vi "sumLinesIntoVolume.vi"(8 "error in (no error)":errorcluster, 10 "volumes to assemble":T3(array[cluster]), 11 "assembler status":T2) -> (0 "error out":errorcluster, 2 "volumes to send":T1(array[cluster]), 3 "assembler status out":T2)   [LabVIEW 2010]
uses:
  get write location linear fit.vi
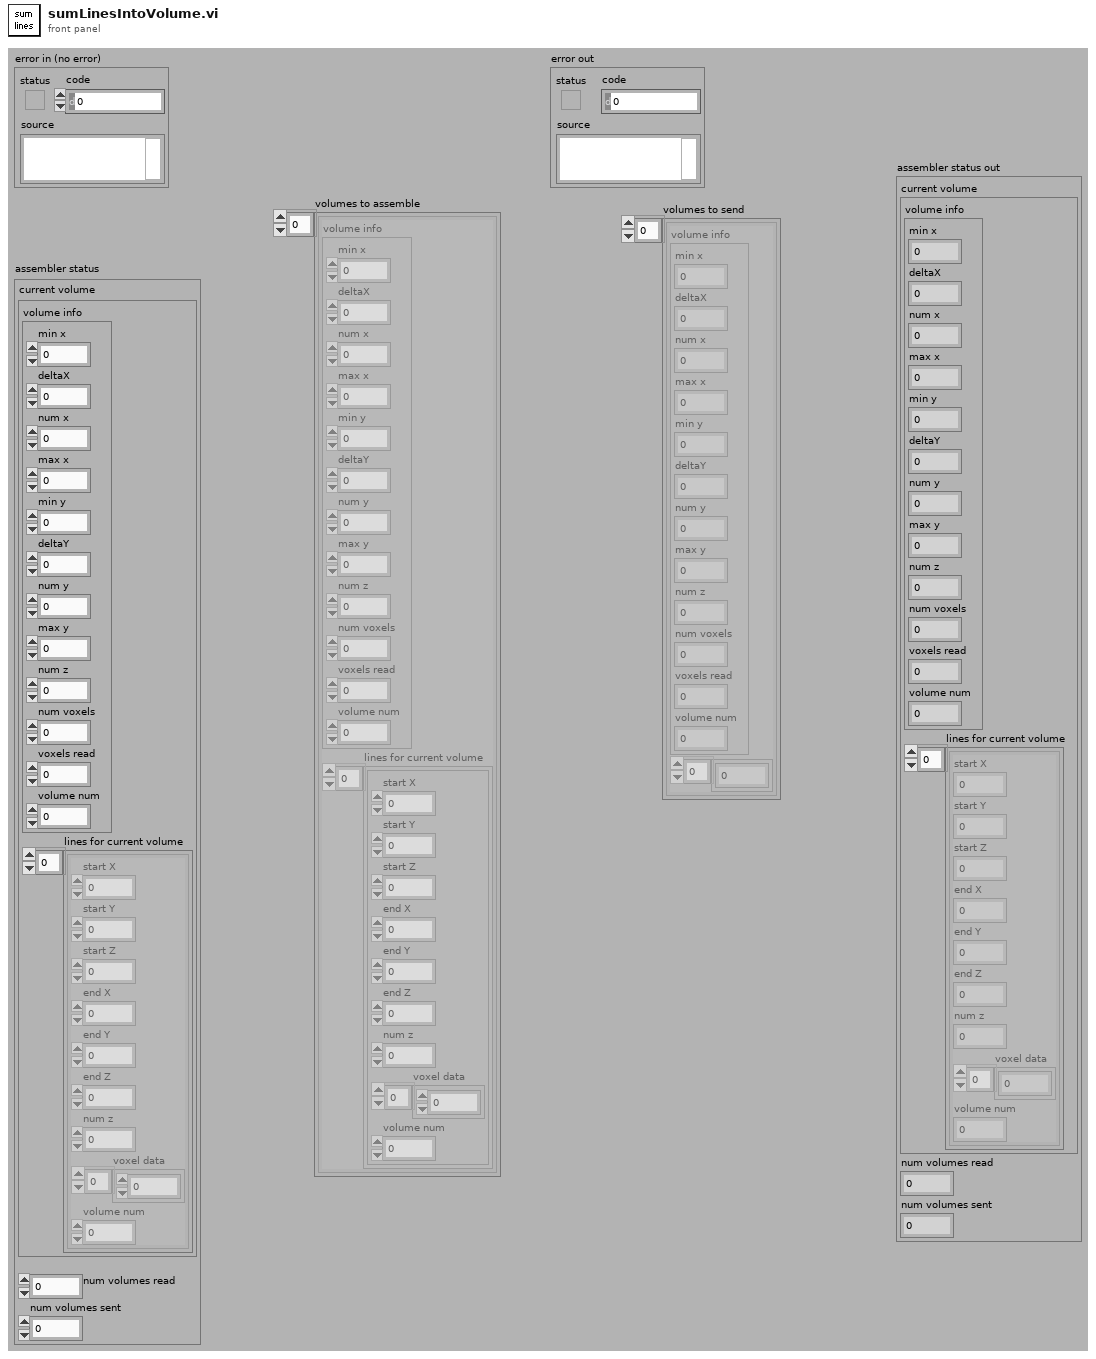
[diagram p1: front panel]
types:
  T1 = cluster{"volume info":cluster{"min x":i16, "deltaX":dbl, "num x":u32, "max x":i16, "min y":i16, "deltaY":dbl, "num y":u32, "max y":i16, "num z":u32, "num voxels":u32, "voxels read":u32, "volume num":u32}, u32[]}[]
  T2 = cluster{"current volume":cluster{"volume info":cluster{"min x":i16, "deltaX":dbl, "num x":u32, "max x":i16, "min y":i16, "deltaY":dbl, "num y":u32, "max y":i16, "num z":u32, "num voxels":u32, "voxels read":u32, "volume num":u32}, "lines for current volume":cluster{"start X":i16, "start Y":i16, "start Z":i16, "end X":i16, "end Y":i16, "end Z":i16, "num z":u8, "voxel data":u32[], "volume num":u32}[]}, "num volumes read":u32, "num volumes sent":u32}
  T3 = cluster{"volume info":cluster{"min x":i16, "deltaX":dbl, "num x":u32, "max x":i16, "min y":i16, "deltaY":dbl, "num y":u32, "max y":i16, "num z":u32, "num voxels":u32, "voxels read":u32, "volume num":u32}, "lines for current volume":cluster{"start X":i16, "start Y":i16, "start Z":i16, "end X":i16, "end Y":i16, "end Z":i16, "num z":u8, "voxel data":u32[], "volume num":u32}[]}[]
  T4 = cluster{"min x":i16, "deltaX":dbl, "num x":u32, "max x":i16, "min y":i16, "deltaY":dbl, "num y":u32, "max y":i16, "num z":u32, "num voxels":u32, "voxels read":u32, "volume num":u32}
  T5 = cluster{"start X":i16, "start Y":i16, "start Z":i16, "end X":i16, "end Y":i16, "end Z":i16, "num z":u8, "voxel data":u32[], "volume num":u32}[]
  T6 = cluster{"volume info":cluster{"min x":i16, "deltaX":dbl, "num x":u32, "max x":i16, "min y":i16, "deltaY":dbl, "num y":u32, "max y":i16, "num z":u32, "num voxels":u32, "voxels read":u32, "volume num":u32}, u32[]}
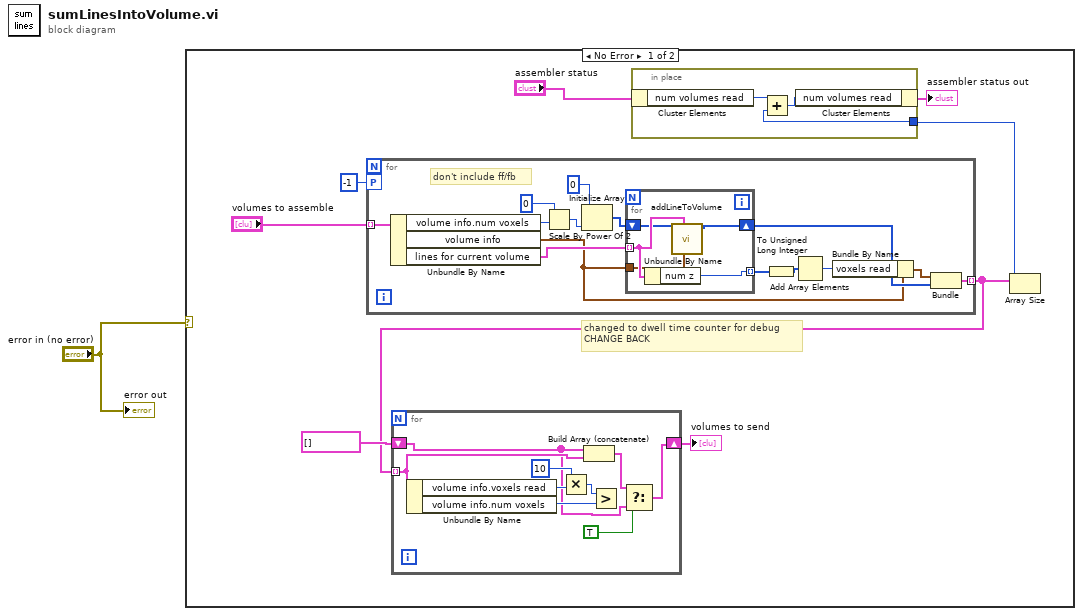
[diagram p0: block diagram]
diagram:
  n1 = case shown="No Error" "error in (no error)" {
    frame No Error {
      # "changed to dwell time counter for debug\nCHANGE BACK"
      n2 = for {
        tunnel: "volumes to assemble" -> [w35] mode=indexing
        tunnel: [w23] -> w6 mode=indexing
        workers-P: -1 -> [_]
        # "don't include ff/fb"
        n3 = Unbundle By Name(w35) -> ("volume info.num voxels"=w34:u32, "volume info"=w24:T4, "lines for current volume"=w29:T5)
        n4 = Scale By Power Of 2(n=0, x=w34) -> (x*2^n=w32:u32)
        n5 = Initialize Array(u32 0, w32) -> (w30:u32[])
        n6 = for {
          tunnel: w24 -> [w38]
          tunnel: w29 -> [w39] mode=indexing
          shift-right: [w36] -> w25
          shift-left: w30 -> [w37]
          tunnel: [w40] -> w28 mode=indexing
          n7 = Unbundle By Name(w39) -> ("num z"=w40:u8)
          n8 = call "addLineToVolume.vi"("current volume"=w38, "line"=w39, "volume buffer"=w37) -> ("volume buffer out"=w36:u32[])  [unwired: 7 in, 1 out]
        }
        n9 = To Unsigned Long Integer(number=w28) -> (unsigned 32bit integer=w22:u32[])
        n10 = Add Array Elements(numeric array=w22) -> (sum=w27:u32)
        n11 = Bundle By Name(cluster=w24, "voxels read"=w27) -> (w26:T4)
        n12 = Bundle("volume info"=w26, w25) -> (w23:T6)  [unwired: 1 in]
      }
      n13 = for {
        tunnel: w6 -> [w17] mode=indexing
        shift-right: [w15] -> w3
        shift-left: T1 [] -> [w14]
        n14 = Unbundle By Name(w17) -> ("volume info.voxels read"=w21:u32, "volume info.num voxels"=w18:u32)
        n15 = Multiply(x=u32 10, y=w21) -> (x*y=w19:u32)
        n16 = Build Array (concatenate)(w14, w17) -> (w16:T1)
        n17 = Greater?(x=w19, y=w18) -> ()  [unwired: 1 out]
        n18 = Select(t=w16, s=TRUE, f=w14) -> (s? t:f=w15:T1)
      }
      "volumes to send" <- w3
      n19 = Array Size(array=w6) -> (size(s)=w5:i32)
      n20 = in-place {
        in-place-border: w5 -> [w11]
        n21 = in-place-cluster #1("assembler status") -> ("num volumes read"=w12:u32)
        n22 = Add(x=w12, y=w11) -> (x+y=w10:u32)
        n23 = in-place-cluster #1("num volumes read"=w10) -> (→"assembler status out":T2)
      }
    }
    frame Error {
    }
  }
  "error out" <- "error in (no error)"
